vi "Automation Program.vi"() -> ()   [LabVIEW 2011]
uses:
  <instrlib>/Tektronix DPO MSO 2000 4000 Series/Public/Data/Read (Single Waveform).vi
  <instrlib>/Tektronix DPO MSO 2000 4000 Series/Tektronix DPO MSO 2000 4000 Series.lvlib
panel:
  in  "How many Loops":i32
  out "Power Meter (W)":dbl(knob) scale=0.0..40.0
  in  "Measurement  (0: Period) 4":i32(ring) items=["Period", "Frequency", "Delay", "Rise Time", "Fall Time", "Positive Duty Cycle", "Negative Duty Cycle", "Positive Pulse Width", "Negative Pulse Width", "Burst Width", "Phase", "Positive Overshoot", "Negative Overshoot", "Vpp", "Amplitude", "Voltage High", "Voltage Low", "Voltage Max", "Voltage Min", "Voltage Mean", "Voltage Mean (cycle)", "Voltage RMS", "Voltage RMS (cycle)", "Area", "Cycle Area", "Positive Edge Count", "Negative Edge Count", "Positive Pulse Count", "Negative Pulse Count"]
  out "Power RMS  (W)":dbl
  out "Voltage":dbl
  in  "Channel2 Voltage":u16(ring) items=["Channel 1", "Channel 2", "Channel 3", "Channel 4", "Math", "Reference 1", "Reference 2", "Reference 3", "Reference 4", "D0", "D1", "D2", "D3", "D4", "D5", "D6", "D7", "D8", "D9", "D10", "D11", "D12", "D13", "D14", "D15", "Amplitude", "Frequency", "Phase", "Normal", "Average", "Maximum Peak Hold", "Minimum Peak Hold"]
  in  "Measurement  3":i32(ring) items=["Period", "Frequency", "Delay", "Rise Time", "Fall Time", "Positive Duty Cycle", "Negative Duty Cycle", "Positive Pulse Width", "Negative Pulse Width", "Burst Width", "Phase", "Positive Overshoot", "Negative Overshoot", "Vpp", "Amplitude", "Voltage High", "Voltage Low", "Voltage Max", "Voltage Min", "Voltage Mean", "Voltage Mean (cycle)", "Voltage RMS", "Voltage RMS (cycle)", "Area", "Cycle Area", "Positive Edge Count", "Negative Edge Count", "Positive Pulse Count", "Negative Pulse Count"]
  out "Measurement Value 3":dbl
  in  "Measurement  2":i32(ring) items=["Period", "Frequency", "Delay", "Rise Time", "Fall Time", "Positive Duty Cycle", "Negative Duty Cycle", "Positive Pulse Width", "Negative Pulse Width", "Burst Width", "Phase", "Positive Overshoot", "Negative Overshoot", "Vpp", "Amplitude", "Voltage High", "Voltage Low", "Voltage Max", "Voltage Min", "Voltage Mean", "Voltage Mean (cycle)", "Voltage RMS", "Voltage RMS (cycle)", "Area", "Cycle Area", "Positive Edge Count", "Negative Edge Count", "Positive Pulse Count", "Negative Pulse Count"]
  out "Measurement Value 2":dbl
  out "Measurement Value 1":dbl
  out "Waveform Graph":waveform(dbl)(graph)
  in  "Measurement  1":i32(ring) items=["Period", "Frequency", "Delay", "Rise Time", "Fall Time", "Positive Duty Cycle", "Negative Duty Cycle", "Positive Pulse Width", "Negative Pulse Width", "Burst Width", "Phase", "Positive Overshoot", "Negative Overshoot", "Vpp", "Amplitude", "Voltage High", "Voltage Low", "Voltage Max", "Voltage Min", "Voltage Mean", "Voltage Mean (cycle)", "Voltage RMS", "Voltage RMS (cycle)", "Area", "Cycle Area", "Positive Edge Count", "Negative Edge Count", "Positive Pulse Count", "Negative Pulse Count"]
  in  "Channel (0: Channel 1)":u16(ring) items=["Channel 1", "Channel 2", "Channel 3", "Channel 4", "Math", "Reference 1", "Reference 2", "Reference 3", "Reference 4", "D0", "D1", "D2", "D3", "D4", "D5", "D6", "D7", "D8", "D9", "D10", "D11", "D12", "D13", "D14", "D15", "Amplitude", "Frequency", "Phase", "Normal", "Average", "Maximum Peak Hold", "Minimum Peak Hold"]
  in  "VISA resource name":refnum<visa-resource-name>
  out "stripped path":path
  out "error out":errorcluster
  in  "Team (eg. Instrumentation)":string
  in  "Name (First and Last)":string
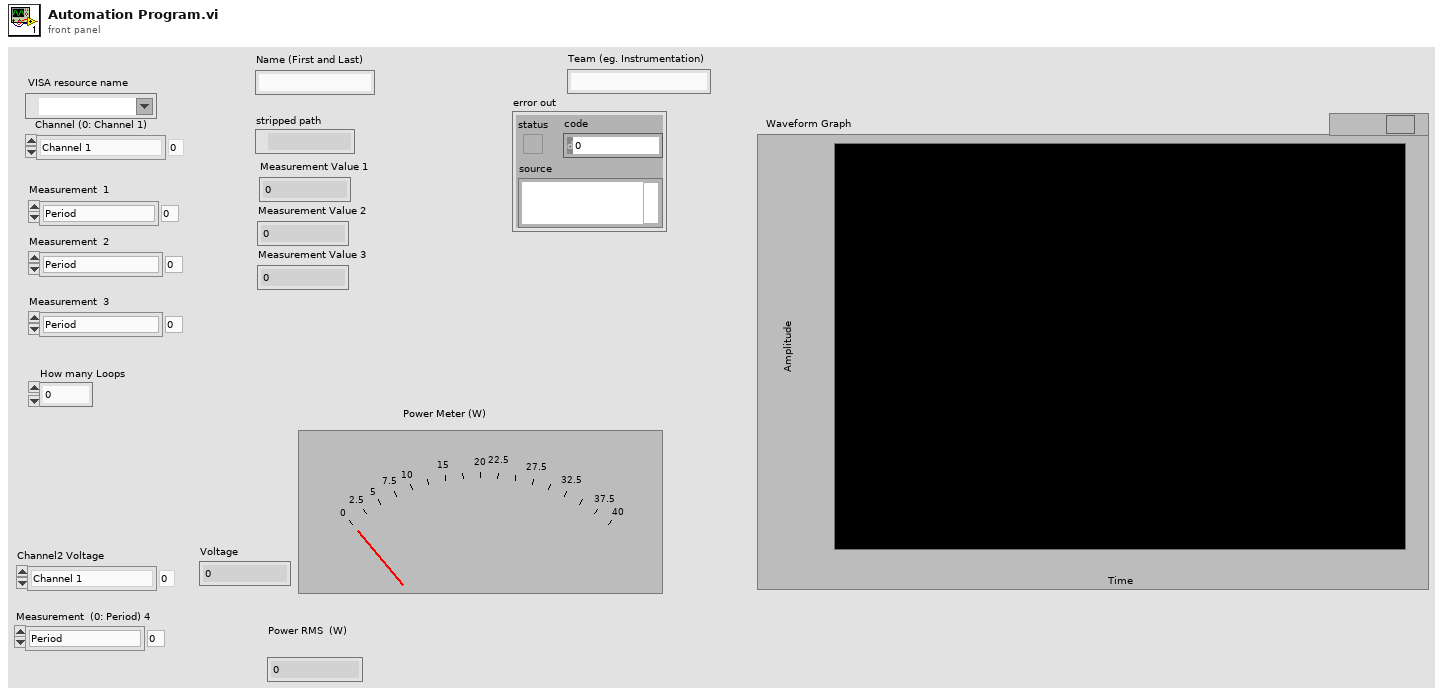
[diagram p1: front panel]
types:
  T1 = enum16{"open", "replace", "create", "open or create", "replace or create", "replace or create with confirmation"}
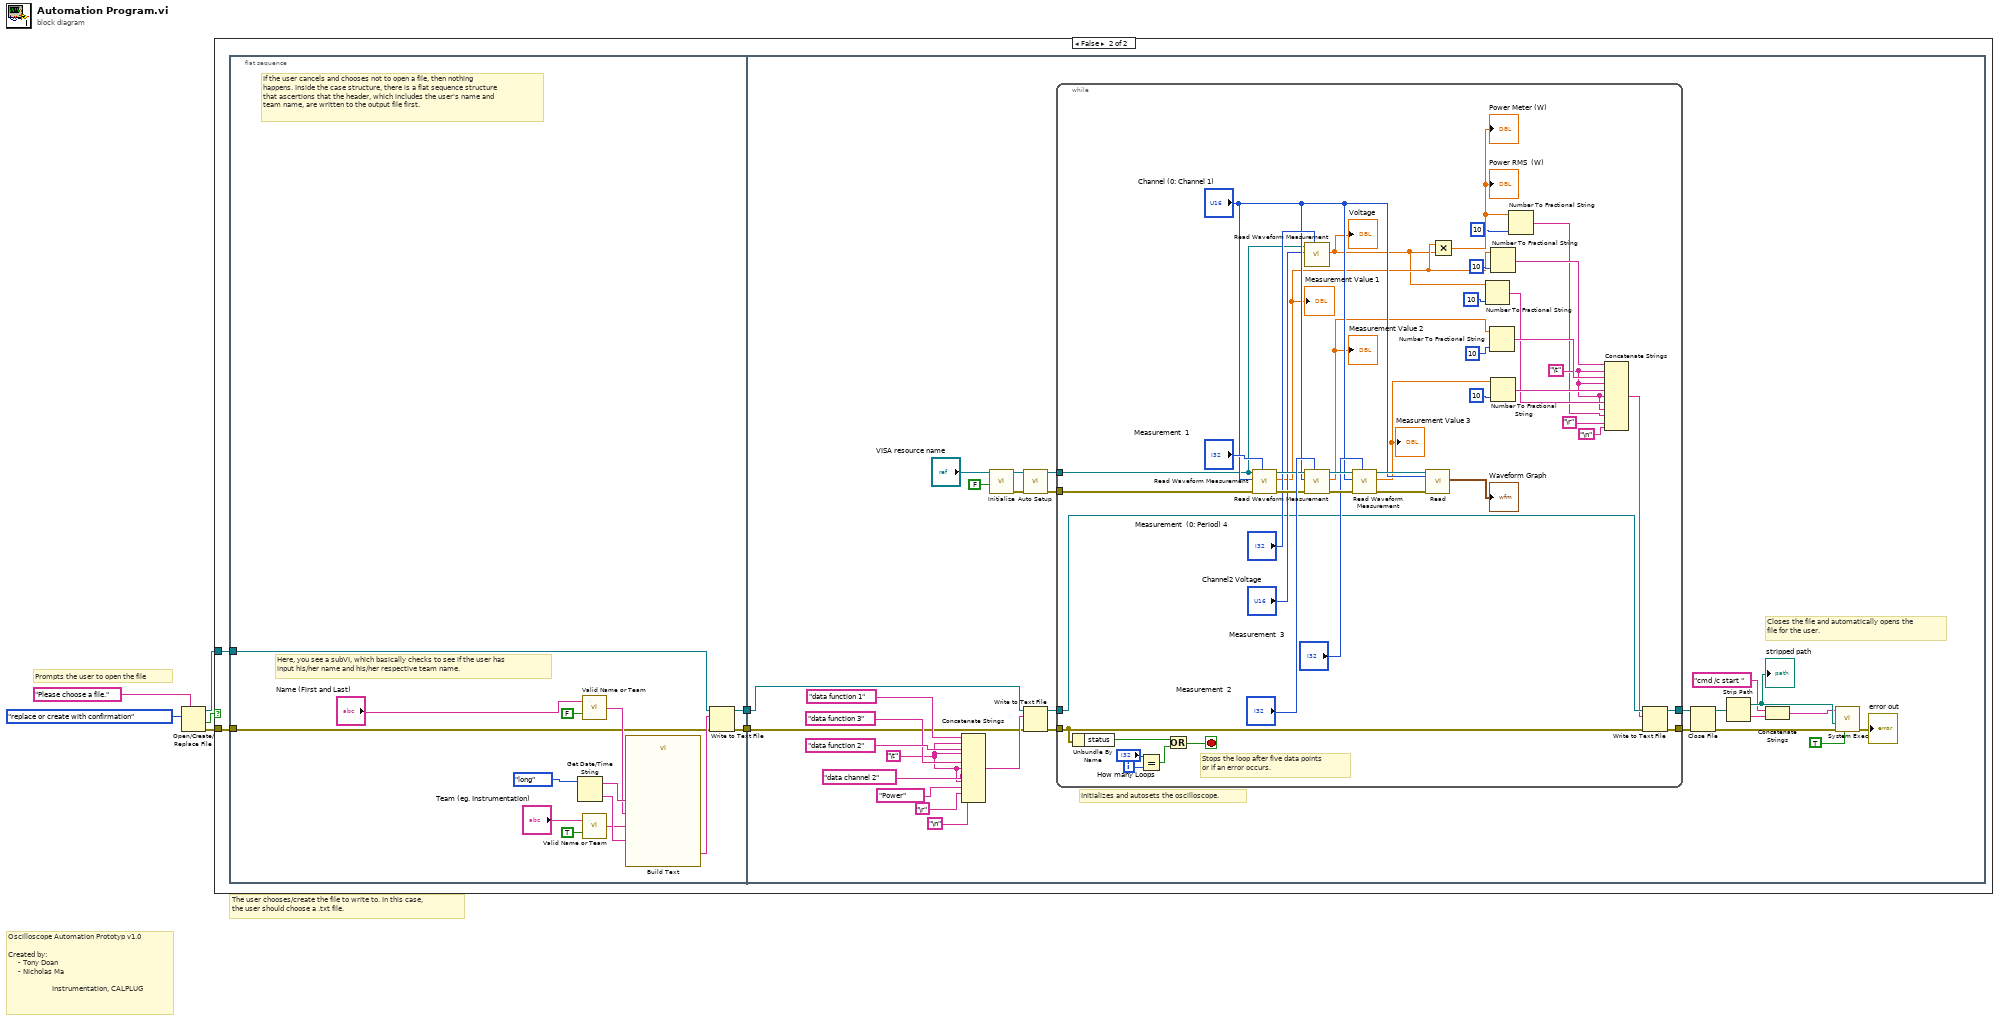
[diagram p0: block diagram]
diagram:
  # "The user chooses/create the file to write to. In this case, \nthe user should choose a .txt file."
  # "Oscilloscope Automation Prototyp v1.0\n\nCreated by:\n     - Tony Doan\n     - Nicholas Ma\n\n                      Instrumentation, CALPLUG"
  # "Prompts the user to open the file"
  n1 = Open/Create/Replace File(prompt="Please choose a file.", operation (0:open)=T1."replace or create with confirmation") -> (refnum out=w2:refnum<file>, cancelled=w3:bool, error out=w1:errorcluster)  [unwired: 4 in]
  n2 = case shown="False" w3 {
    tunnel: w2 -> [_ w8]
    tunnel: w1 -> [_ w9]
    frame True {
    }
    frame False {
      n3 = flat-sequence {
        tunnel: w9 -> [w13]
        tunnel: w8 -> [w12]
        tunnel: [w11] -> w7
        tunnel: [w10] -> w6
        tunnel: w7 -> [w38]
        tunnel: w6 -> [w32]
        frame #0 {
          # "Here, you see a subVI, which basically checks to see if the user has\ninput his/her name and his/her respective team name."
          # "If the user cancels and chooses not to open a file, then nothing\nhappens. Inside the case structure, there is a flat sequence structure\nthat ascertions that the header, which includes the user's name and\nteam name, are written to the output file first."
          n4 = Get Date/Time String(date format (0)=enum16{"short", "long", "abbreviated"}."long") -> (date string=w21:string, time string=w22:string)  [unwired: 2 in]
          n5 = call "Valid Name or Team.vi"("Input Boolean"=FALSE, "Input String"="Name (First and Last)") -> ("Output String"=w19:string)
          n6 = call "Valid Name or Team.vi"("Input Boolean"=TRUE, "Input String"="Team (eg. Instrumentation)") -> ("Output String"=w20:string)
          n7 = call "Build Text"("Time"=w22, "Name"=w19, "Team"=w20, "Date"=w21) -> ("Result"=w23:string)  [unwired: 10 in, 1 out]
          n8 = Write to Text File(file (use dialog)=w12, text=w23, error in=w13) -> (refnum out=w11:refnum<file>, error out=w10:errorcluster)  [unwired: 1 in, 1 out]
        }
        frame #1 {
          w27 = "\t"
          # "Closes the file and automatically opens the\nfile for the user."
          # "Initializes and autosets the oscilloscope."
          n9 = Concatenate Strings("data function 1" ("string"), w27, "data function 2" ("string"), w27, "data function 3" ("string"), w27, "data channel 2" ("string"), w27, "Power" ("string"), "\r", "\n") -> (w34:string)
          n10 = call <instrlib>:"Initialize.vi"("Reset (True)"=FALSE, "VISA resource name"="VISA resource name") -> ("error out"=w44:errorcluster, "VISA resource name out"=w43:refnum<visa-resource-name>)  [unwired: 8 in]
          n11 = call <instrlib>:"Auto Setup.vi"("error in (no error)"=w44, "VISA resource name"=w43) -> ("error out"=w39:errorcluster, "VISA resource name out"=w40:refnum<visa-resource-name>)  [unwired: 8 in]
          n12 = Write to Text File(file (use dialog)=w38, text=w34, error in=w32) -> (refnum out=w33:refnum<file>, error out=w31:errorcluster)  [unwired: 1 in, 1 out]
          n13 = while {
            tunnel: w40 -> [w82]
            tunnel: w39 -> [w81]
            tunnel: w33 -> [w80]
            tunnel: w31 -> [w69]
            tunnel: [w72] -> w30
            tunnel: [w71] -> w29
            i -> [w70]
            stop <- w67 stop-if-true
            w57 = "\t"
            # "Stops the loop after five data points\nor if an error occurs."
            n14 = Unbundle By Name(w69) -> ("status"=w68:bool)
            n15 = Equal?(x="How many Loops", y=w70) -> (x = y?=w66:bool)
            n16 = Or(x=w68, y=w66) -> (x .or. y?=w67:bool)
            n17 = call <instrlib>:"Read Waveform Measurement.vi"("Measurement Function (0: Period)"="Measurement  1", "error in (no error)"=w81, "Channel (0: Channel 1)"="Channel (0: Channel 1)", "VISA resource name"=w82) -> ("error out"=w92:errorcluster, "Measurement Value"=w59:dbl, "VISA resource name out"=w90:refnum<visa-resource-name>)  [unwired: 5 in]
            "Measurement Value 1" <- w59
            n18 = call <instrlib>:"Read Waveform Measurement.vi"("Measurement Function (0: Period)"="Measurement  (0: Period) 4", "Channel (0: Channel 1)"="Channel2 Voltage", "VISA resource name"=w82) -> ("Measurement Value"=w53:dbl)  [unwired: 6 in, 2 out]
            "Voltage" <- w53
            n19 = call <instrlib>:"Read Waveform Measurement.vi"("Measurement Function (0: Period)"="Measurement  2", "error in (no error)"=w92, "Channel (0: Channel 1)"="Channel (0: Channel 1)", "VISA resource name"=w90) -> ("error out"=w91:errorcluster, "Measurement Value"=w78:dbl, "VISA resource name out"=w89:refnum<visa-resource-name>)  [unwired: 5 in]
            "Measurement Value 2" <- w78
            n20 = call <instrlib>:"Read Waveform Measurement.vi"("Measurement Function (0: Period)"="Measurement  3", "error in (no error)"=w91, "Channel (0: Channel 1)"="Channel (0: Channel 1)", "VISA resource name"=w89) -> ("error out"=w87:errorcluster, "Measurement Value"=w76:dbl, "VISA resource name out"=w88:refnum<visa-resource-name>)  [unwired: 5 in]
            "Measurement Value 3" <- w76
            n21 = call-poly <instrlib>:"Read.vi"("error in (no error)"=w87, "Channel (0: Channel 1)"="Channel (0: Channel 1)", "VISA resource name"=w88) -> ("Waveform Graph"=→"Waveform Graph":waveform(dbl))  [unwired: 6 in, 2 out]
            n22 = Multiply(x=w59, y=w53) -> (x*y=w74:dbl)
            "Power RMS  (W)" <- w74
            "Power Meter (W)" <- w74
            n23 = Number To Fractional String(number=w53, precision (6)=i16 10 ("width (-)")) -> (F-format string=w58:string)  [unwired: 2 in]
            n24 = Number To Fractional String(number=w78, precision (6)=i16 10 ("width (-)")) -> (F-format string=w77:string)  [unwired: 2 in]
            n25 = Number To Fractional String(number=w59, precision (6)=i16 10 ("width (-)")) -> (F-format string=w79:string)  [unwired: 2 in]
            n26 = Number To Fractional String(number=w76, precision (6)=i16 10 ("width (-)")) -> (F-format string=w75:string)  [unwired: 2 in]
            n27 = Number To Fractional String(number=w74, precision (6)=i16 10 ("width (-)")) -> (F-format string=w56:string)  [unwired: 2 in]
            n28 = Concatenate Strings(w79, w57, w77, w57, w75, w57, w58, w57, w56, "\r", "\n") -> (w73:string)
            n29 = Write to Text File(file (use dialog)=w80, text=w73, error in=w69) -> (refnum out=w72:refnum<file>, error out=w71:errorcluster)  [unwired: 1 in, 1 out]
          }
          n30 = Close File(refnum=w30, error in=w29) -> (path=w48:path, error out=w51:errorcluster)
          n31 = Strip Path(path=w48) -> (stripped path=w50:path, name=w49:string)
          "stripped path" <- w50
          n32 = Concatenate Strings("cmd /c start " ("string"), w49) -> (w47:string)
          n33 = call <vilib>:"System Exec.vi"("run minimized? (F)"=TRUE, "error in (no error)"=w51, "working directory"=w50, "command line"=w47) -> ("error out"=→"error out":errorcluster)  [unwired: 4 in, 3 out]
        }
      }
    }
  }
